vi "Convert Node Result to Test Suite - Specified Registration Call Chain - Package is Registration Call Chain Library Name.vi"() -> ()   [LabVIEW 2013, in "JUnit Conversion Tests.lvlib"]
uses:
  JUnit Conversion Tests.lvlib
  <vilib>/addons/_JKI Toolkits/Caraya/classes/Test Result/Node Results (Extended).ctl
  <vilib>/addons/_JKI Toolkits/Caraya/classes/Test Result/Test Node (Extended).ctl
  <vilib>/addons/_JKI Toolkits/Caraya/classes/Test Result/Test Registration Data.ctl
  <vilib>/addons/_JKI Toolkits/Caraya/classes/Test Result/Assert Event Data (Extended).ctl
  <vilib>/addons/_JKI Toolkits/Caraya/classes/MsgSerializer/MsgSerializer.lvclass
  JUnit XML/Test Suite/Test Suite.lvclass/Test Suite.ctl
  JUnit XML/Test Suite/Read Package.vi
  <vilib>/addons/_JKI Toolkits/Caraya/classes/Assert/Assert Equal Value_Variant.vi
  <vilib>/addons/_JKI Toolkits/Caraya/classes/Assert/Assert.lvclass
  <vilib>/addons/_JKI Toolkits/Caraya/classes/Test/Test.lvclass
  JUnit Conversion/JUnit Conversion.lvlib
  <vilib>/addons/_JKI Toolkits/Caraya/classes/Test Result/Test Result.lvclass
  JUnit XML/Test Suite/Test Suite.lvclass
panel:
  out "error out":errorcluster
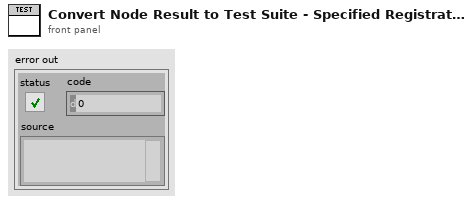
[diagram p1: front panel]
types:
  T1 = typedef "Caraya.lvlib/Test Result.lvclass/Node Results (Extended).ctl" = cluster{"Test Node":T2, "Assertions":T4[]}
  T2 = typedef "Caraya.lvlib/Test Result.lvclass/Test Node (Extended).ctl" = cluster{"Test Registration":T3, "Defined":bool, "Passed":bool, "properties":variant}
  T3 = typedef "Caraya.lvlib/Test Result.lvclass/Test Registration Data.ctl" = cluster{"Name":string, "Call Chain":string[], "Time Stamp":timestamp, "Test ID":string, "Caller ID":string}
  T4 = typedef "Caraya.lvlib/Test Result.lvclass/Assert Event Data (Extended).ctl" = cluster{"name":string, "passed":bool, "call-chain":string[], "test-error":errorcluster, "timestamp":timestamp, "assert-id":string, "test-id":string, "time":dbl, "message":string, "properties":variant, "measurements":variant, "user-defined":variant}
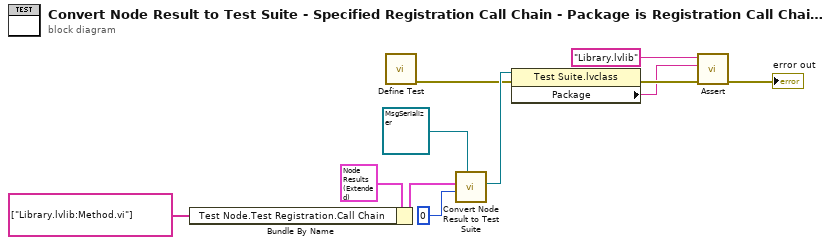
[diagram p0: block diagram]
diagram:
  n1 = Bundle By Name(cluster=T1 {"Test Node"={"Test Registration"={"Name"="", "Call Chain"=[], "Time Stamp"=timestamp(0 s since 1904-01-01), "Test ID"="", "Caller ID"=""}, "Defined"=FALSE, "Passed"=FALSE, "properties"=variant}, "Assertions"=[]} ("Node Result"), "Test Node.Test Registration.Call Chain"=string[] ["Library.lvlib:Method.vi"]) -> (w3:T1)
  n2 = call <vilib>:"Define Test.vi"() -> ("error out"=w8:errorcluster)  [unwired: 10 in, 1 out]
  n3 = call "Convert Node Result to Test Suite.vi"("MsgSerializer"=refnum<class "MsgSerializer.lvclass"> refnum, "ID"=0, "Node Result"=w3) -> ("Test Suite"=w11:refnum<class "Test Suite.lvclass">)  [unwired: 8 in]
  n4 = property class="Test Suite.lvclass"(reference=w11, error in=w8) -> (error out=w10:errorcluster, "Package"=w9:string)  [unwired: 1 out]
  n5 = call-poly <vilib>:"Assert.vi"("error in (no error)"=w10, "Y"=w9, "X"="Library.lvlib") -> ("error out"=→"error out":errorcluster)  [unwired: 7 in, 1 out]
